vi "demodulate_all.vi"(6 "Config":T5={"IO params"={"Conversion"={"Rate"=4.0, "Num cards"=2, "Out channels"=4}, "Carriers"={"Phase shift"=180.0, "Levels"=[[0.8, 0.8, 0.8], [0.03, 0.03, 0.03]], "Delay samples"=73.15}, "TCP"={"Host"="192.168.1.15", "Port"=6666, "Buffering"=6, "Timeout"=6}, "Input channel sign"=[1, 1, 1]}, "High rate STFT"={"Win param"=101.5, "Window type"=61, "Win order"=2, "DFT size"=64, "Channels"=[7], "Oversample"=64}, "Low rate STFT"={"Win param"=120.0, "Window type"=61, "Win order"=8, "DFT size"=64, "Channels"=[7], "Oversample"=64}, "Filtering "=[]} {"Filtering"."Distortion"."Limit" format="%#_3p"; "Filtering"."Distortion"."LF cut" format="%#_3p"; "Filtering"."Kalman"."Measure noise" format="%#_3p"; "Filtering"."Kalman"."Process noise" format="%#_3p"; "Filtering"."Hum"."Limit" format="%#_3p"; "Filtering"."Hum"."Frequency" format="%#_4p"; "Low rate STFT"."Oversample" min=1 step=1; "Low rate STFT"."Channels" min=0 step=1; "Low rate STFT"."DFT size" min=1 step=1; "Low rate STFT"."Window type" items=["Rectangle"=0, "Hanning"=1, "Hamming"=2, "Blackman-Harris"=3, "Exact Blackman"=4, "Blackman"=5, "Flat Top"=6, "4 Term B-Harris "=7, "7 Term B-Harris"=8, "Low Sidelobe"=9, "Blackman Nuttall"=11, "Triangle"=30, "Bartlett-Hanning"=31, "Bohman"=32, "Parzen"=33, "Welch"=34, "Kaiser"=60, "Dolph-Chebyshev"=61, "Gaussian"=62]; "High rate STFT"."Oversample" min=1 step=1; "High rate STFT"."Channels" min=0 step=1; "High rate STFT"."DFT size" min=1 step=1; "High rate STFT"."Window type" items=["Rectangle"=0, "Hanning"=1, "Hamming"=2, "Blackman-Harris"=3, "Exact Blackman"=4, "Blackman"=5, "Flat Top"=6, "4 Term B-Harris "=7, "7 Term B-Harris"=8, "Low Sidelobe"=9, "Blackman Nuttall"=11, "Triangle"=30, "Bartlett-Hanning"=31, "Bohman"=32, "Parzen"=33, "Welch"=34, "Kaiser"=60, "Dolph-Chebyshev"=61, "Gaussian"=62]; "IO params"."Input channel sign" min=-1 max=1 step=1; "IO params"."Carriers"."Levels" min=0.0 step=0.1; "IO params"."Conversion"."Rate" format="%#_8g"}, 7 "Prev carrier amplitudes":T12 format="%#_3p", 8 "Input card":i32=1, 9 "Modulation info":T4 {"Hi channels at low" min=0 step=1; "Low carriers" format="%#_6p"; "High carriers" format="%#_6p"}, 10 "Reset":bool, 11 "Raw data":dbl[][][](array[numeric])) -> (2 "Trace info out":T1, 3 "High carrier amplitudes":T11 format="%#_3p", 5 "NaN":bool)   [LabVIEW 2026]
uses:
  carrier_amplitudes.ctl
  high_carrier_amplitudes.ctl
  ilemt_config.ctl
  system/IO_params.ctl
  stft_params.ctl
  <vilib>/Analysis/4window.llb/windowTd.ctl
  filter_params.ctl
  detrend_mode.ctl
  modulation_info.ctl
  gui/trace_info.ctl
  gui/trace_channel.ctl
  main/ilemt_status.ctl
  <vilib>/Analysis/NI_AALPro.lvlib
panel:
  # "Carrier amplitudes from previous low-rate measurement cycle.  Our interest is with the low carriers, but the whole deal is passed here.  See demod_low.vi for description of carrier amplitudes"
  # "The carrier amplitudes at the high output rate.  This is a bunch of coupling matrices, grouped by input card and sample index."
  # "Page is the input card number, where current sense is card 0, and later cards are for sensors.  The row is XYZ and the column is sample."
  # "Card"
  # "XYZ In channel"
  # "Full rate sample"
  # "High rate demodulation for all of the cards and input channels.  For now, only demodulate card 0 (current sense) and \"Input card\".  These appear as cards 0 and 1 in the output."
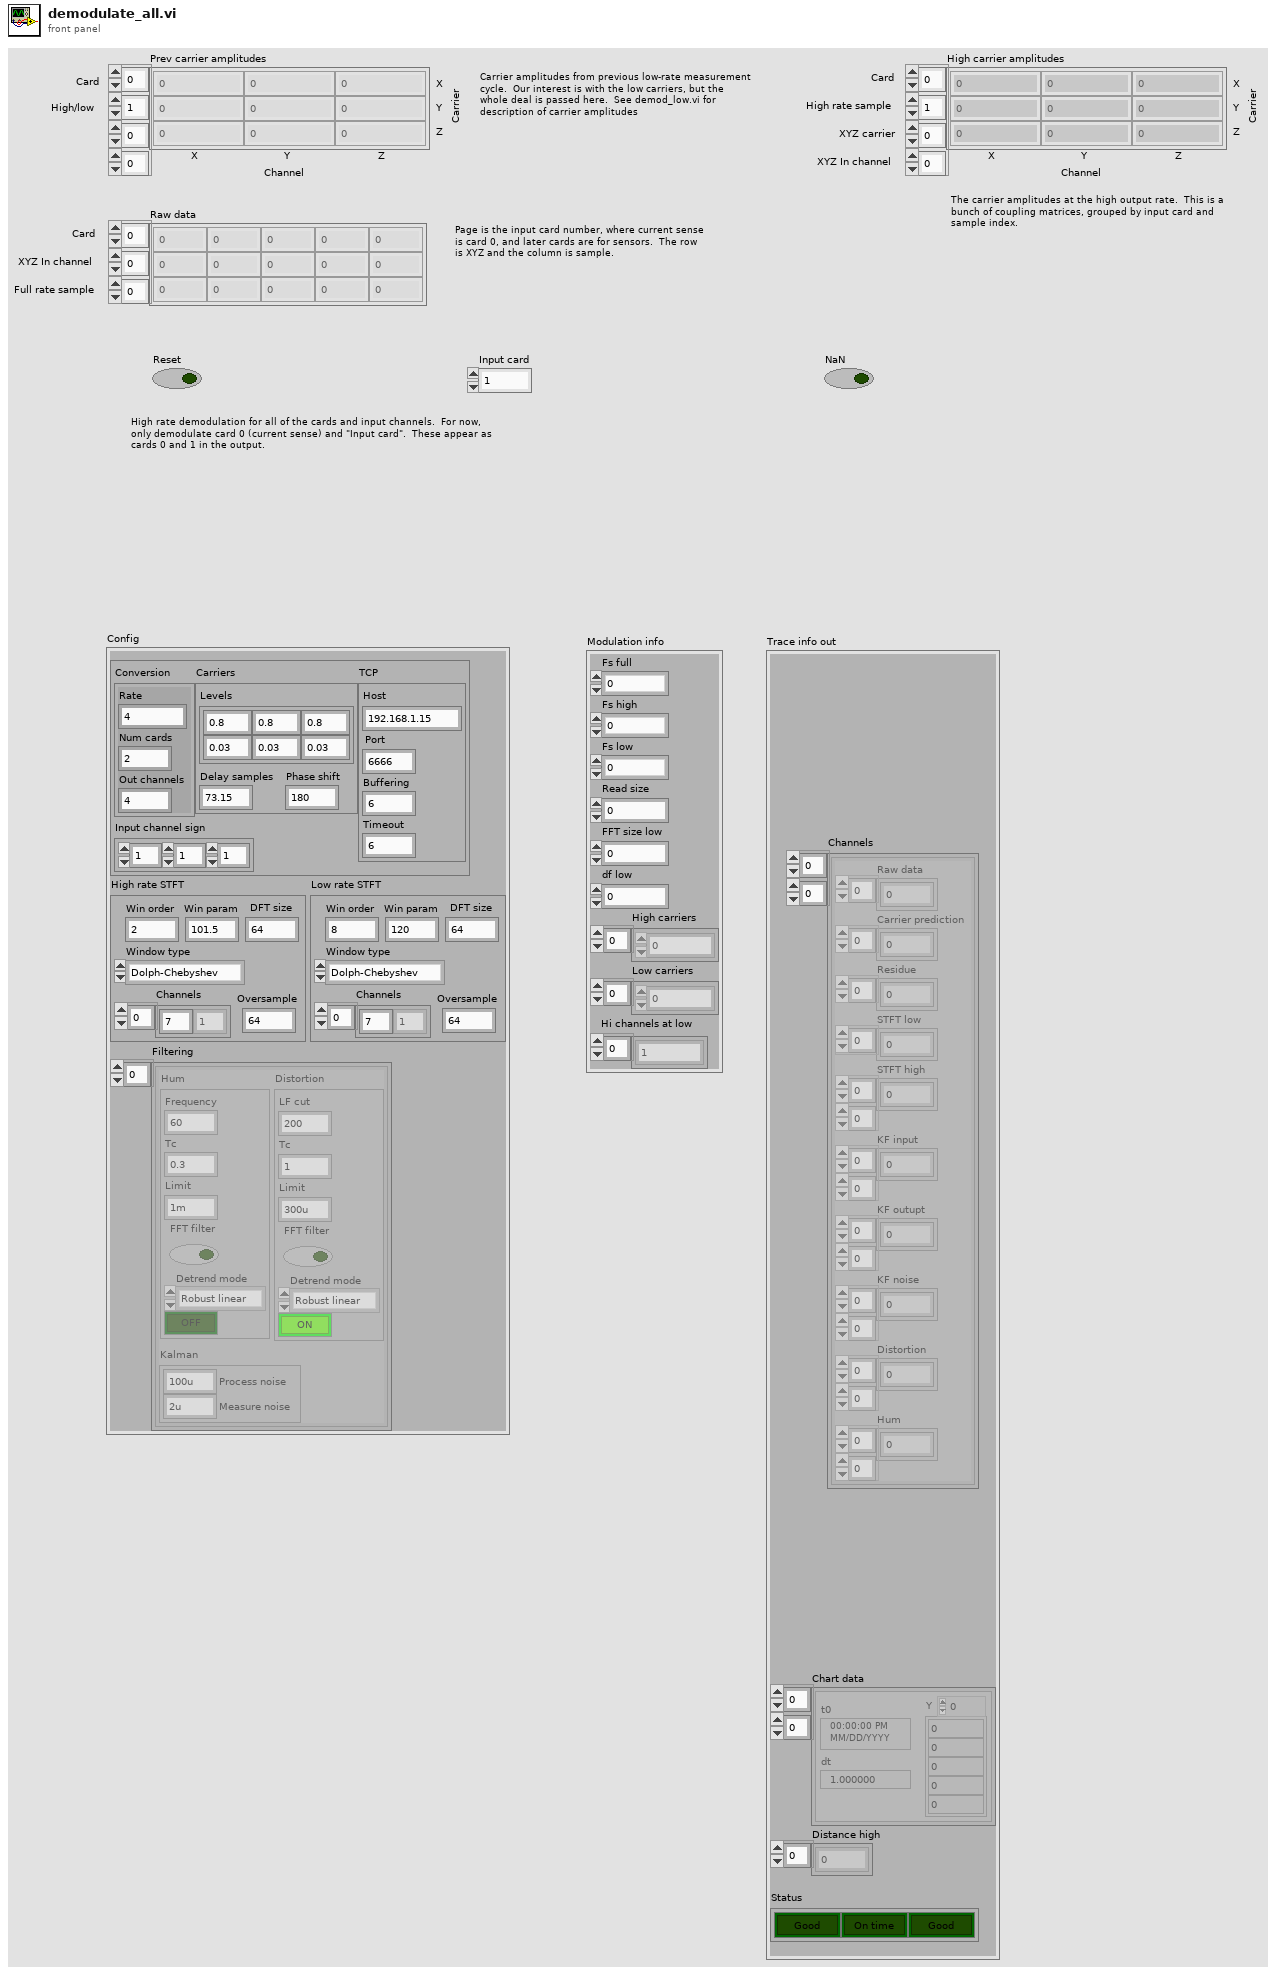
[diagram p1: front panel]
types:
  T1 = typedef "trace_info.ctl" = cluster{"Channels":T2[][], "Chart data":waveform(dbl)[][], "Distance high":dbl[], "Status":T3}
  T2 = typedef "trace_channel.ctl" = cluster{"Raw data":dbl[], "Carrier prediction":dbl[], "Residue":dbl[], "STFT low":cdb[], "STFT high":cdb[][], "KF input":cdb[][], "KF outupt":cdb[][], "KF noise":dbl[][], "Distortion":cdb[][], "Hum":cdb[][]}
  T3 = typedef "ilemt_status.ctl" = cluster{"NaN":bool, "Backlog":bool, "Clipping":bool}
  T4 = typedef "modulation_info.ctl" = cluster{"Fs full":dbl, "Fs high":dbl, "Fs low":dbl, "Read size":i32, "FFT size low":i32, "df low":dbl, "High carriers":dbl[], "Low carriers":dbl[], "Hi channels at low":i32[]}
  T5 = typedef "ilemt_config.ctl" = cluster{"IO params":T6, "High rate STFT":T7, "Low rate STFT":T7, "Filtering ":T9[]}
  T6 = typedef "IO_params.ctl" = cluster{"Conversion":cluster{"Rate":dbl, "Num cards":u32, "Out channels":u32}, "Carriers":cluster{"Phase shift":dbl, "Levels":dbl[][], "Delay samples":dbl}, "TCP":cluster{"Host":string, "Port":i32, "Buffering":u32, "Timeout":u32}, "Input channel sign":i32[]}
  T7 = typedef "stft_params.ctl" = cluster{"Win param":dbl, "Window type":T8, "Win order":i32, "DFT size":i32, "Channels":i32[], "Oversample":i32}
  T8 = typedef "NI_AALPro.lvlib/windowTd.ctl" = u32
  T9 = typedef "filter_params.ctl" = cluster{"Hum":cluster{"Frequency":dbl, "Tc":dbl, "Limit":dbl, "FFT filter":bool, "Detrend mode":T10, "Enable":bool}, "Kalman":cluster{"Process noise":dbl, "Measure noise":dbl}, "Distortion":cluster{"LF cut":dbl, "Tc":dbl, "Limit":dbl, "FFT filter":bool, "Detrend mode":T10, "Enable":bool}}
  T10 = typedef "detrend_mode.ctl" = enum16{"Zero mean", "Linear", "Robust linear"}
  T11 = typedef "high_carrier_amplitudes.ctl" = cdb[][][][]
  T12 = typedef "carrier_amplitudes.ctl" = cdb[][][][]
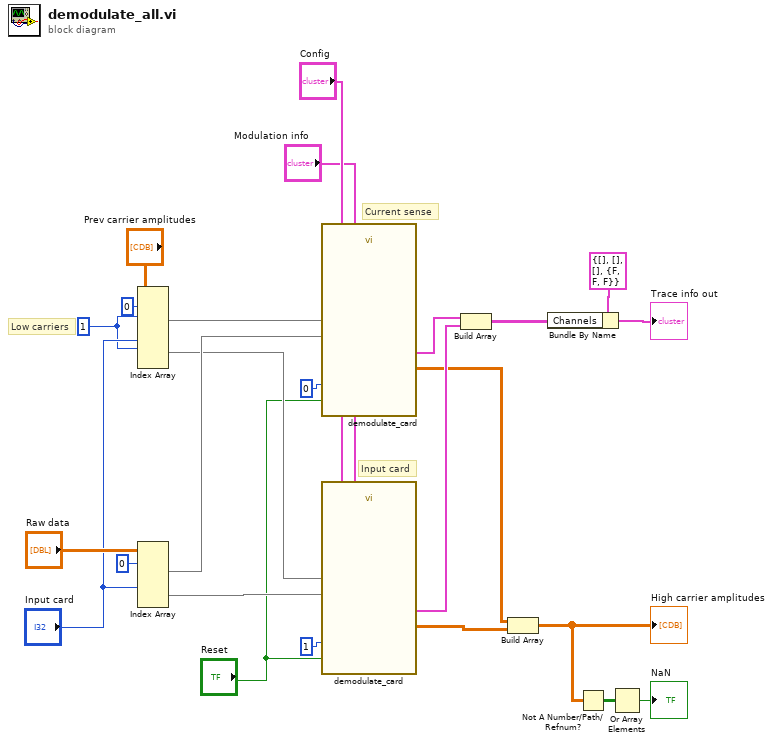
[diagram p0: block diagram]
diagram:
  w7 = 1 ("disabled index (page)")
  # "Input card"
  # "Current sense"
  # "Low carriers"
  n1 = Index Array(array="Prev carrier amplitudes", index (dim 0) #1=0 ("disabled index (vol)"), index (dim 1) #1=w7, index (dim 0) #2="Input card", index (dim 1) #2=w7) -> (element #1=w23:cdb[][], element #2=w14:cdb[][])  [unwired: 4 in]
  n2 = Index Array(array="Raw data", index (dim 0) #1=0 ("index (page)"), index (dim 0) #2="Input card") -> (element #1=w18:dbl[][], element #2=w13:dbl[][])  [unwired: 4 in]
  n3 = call "demodulate_card.vi"("Current/sensor index"=0, "Raw data"=w18, "Reset"="Reset", "Low carrier amplitudes"=w23, "Modulation info"="Modulation info", "Config"="Config") -> ("High carrier amplitudes"=w3:cdb[][][], "Trace channels"=w17:T2[])  [unwired: 4 in]
  n4 = call "demodulate_card.vi"("Current/sensor index"=1, "Raw data"=w13, "Reset"="Reset", "Low carrier amplitudes"=w14, "Modulation info"="Modulation info", "Config"="Config") -> ("High carrier amplitudes"=w11:cdb[][][], "Trace channels"=w10:T2[])  [unwired: 4 in]
  n5 = Build Array(w17, w10) -> (w16:T2[][])
  n6 = Build Array(w3, w11) -> (w9:cdb[][][][])
  "High carrier amplitudes" <- w9
  n7 = Bundle By Name(cluster=T1 {"Channels"=[], "Chart data"=[], "Distance high"=[], "Status"={"NaN"=FALSE, "Backlog"=FALSE, "Clipping"=FALSE}} ("Trace info out"), "Channels"=w16) -> (→"Trace info out":T1)
  n8 = Not A Number/Path/Refnum?(number/path/refnum=w9) -> (NaN/Path/Refnum?=w20:bool[][][][])
  n9 = Or Array Elements(Boolean array=w20) -> (logical OR=→"NaN":bool)
